vi "TurnCCW2Target.vi"   [LabVIEW 2016, in "Project 2 LabVIEW.lvrbt"]
uses:
  Project 2 LabVIEW.lvrbt
  <vilib>/NXT/Block Support/NXT_InputPort.ctl
  <vilib>/NXT/Block Support/NXT_OutputPort.ctl
  <vilib>/NXT/Dual Mode Library/Sensors/EV3_Ultrasonic_CM.vi
  <vilib>/NXT/NXTIO Xnodes/NXTIONodeSubVIs/NXTMoveMotors.vi
  <vilib>/NXT/NXTIO Xnodes/AddressXNode/NXTIOAddress.xnode
  <vilib>/NXT/Subs/LVHSConnector.ctl
  <vilib>/NXT/NXTIO Xnodes/NXTIOXNode/NXTIO.xnode
  <vilib>/NXT/LegoClasses/BrickReference/BrickReference.lvclass
types:
  T1 = typedef "NXT_OutputPort.ctl" = u8
  T2 = typedef "NXT_InputPort.ctl" = u32
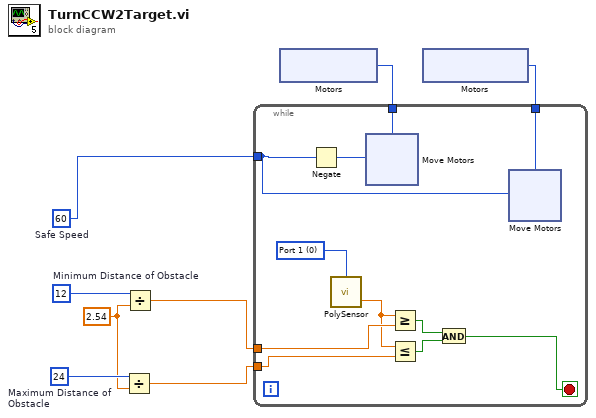
[diagram p0: block diagram]
diagram:
  w3 = 2.54
  w6 = 60  # Safe Speed
  w4 = 24  # Maximum Distance of Obstacle
  w5 = 12  # Minimum Distance of Obstacle
  n1 = Divide(x=w4, y=w3) -> (x/y=w1:dbl)
  n2 = Divide(x=w5, y=w3) -> (x/y=w2:dbl)
  n3 = xnode "Motors"() -> ("Motor"=w8:T1)
  n4 = xnode "Motors"() -> ("Motor"=w7:T1)
  n5 = while {
    tunnel: w8 -> [w19]
    tunnel: w7 -> [w18]
    tunnel: w6 -> [w16]
    tunnel: w2 -> [w11]
    tunnel: w1 -> [w10]
    stop <- w12 stop-if-true
    w15 = T2 0 items=["Port 1", "Port 2", "Port 3", "Port 4"] ("Port (Port 1)")
    n6 = Negate(x=w16) -> (-x=w17:i32)
    n7 = call-poly <vilib>:"PolySensor.vi"("Port (Port 1)"=w15) -> ("Centimeters"=w9:sgl)  [unwired: 2 in, 1 out]
    n8 = xnode "Move Motors"("Power/Speed 1"=w17, "Motors"=w19) -> ()  [unwired: 1 in, 1 out]
    n9 = Greater Or Equal?(x=w9, y=w11) -> (x >= y?=w14:bool)
    n10 = Less Or Equal?(x=w9, y=w10) -> (x <= y?=w13:bool)
    n11 = And(x=w14, y=w13) -> (x .and. y?=w12:bool)
    n12 = xnode "Move Motors"("Power/Speed 1"=w16, "Motors"=w18) -> ()  [unwired: 1 in, 1 out]
  }
